vi "08-QNET_MECHKIT_Magnetic_Field.vi"() -> ()   [LabVIEW 2012]
doc: "This VI is to be used with the NI-ELVIS and the QNET-Mechatronic Sensors I module. The objective is to calibrate the magnetic field sensor."
uses:
  <vilib>/Simulation/Scripting/Companion Diagram/SimConfigNode/SimParams.ctl
  <vilib>/Simulation/Scripting/Companion Diagram/SimConfigNode/_simSolvers.ctl
  <vilib>/Simulation/Implementation/Shared/SIMSCR Execution Mode.ctl
  <vilib>/Simulation/Param Hierarchy/Typedefs/SIMPH Param Control Actions.ctl
  <vilib>/Simulation/Implementation/Shared/NILVSim_ParamChanged.vi
  <vilib>/Simulation/SignalDisplay/Implementation/NILVSim Time Waveform.llb/SIM Time Waveform (scalar).vi
  <vilib>/Simulation/Utility/Implementation/SIM Halt.vi
  <vilib>/Simulation/Implementation/Shared/NILVSim_Manager.vi
  <vilib>/Simulation/Implementation/Shared/NILVSim_FinalizeModel.vi
  <vilib>/Simulation/Implementation/Shared/SIM Unbundle Sim Info.vi
  <vilib>/Utility/error.llb/Clear Errors.vi
  <vilib>/Simulation/Implementation/Shared/NILVSim_GetModelError.vi
  <vilib>/Simulation/Implementation/Shared/SIM Bundle Sim Info.vi
  <vilib>/Simulation/Implementation/Shared/SIMSH Read Queue.vi
  <vilib>/Simulation/Implementation/Shared/NILVSim_Initialize.vi
  <vilib>/Analysis/6fits.llb/Unconstrained Exponential Fit.vi
  <vilib>/DAQmx/read.llb/DAQmx Read.vi
  <vilib>/DAQmx/read.llb/DAQmx Read (Analog DBL 1Chan 1Samp).vi
  <vilib>/Simulation/Utility/Implementation/NILVSim Get Time and IsAcceptedStep.vi
  <vilib>/Simulation/Scripting/Companion Diagram/SimConfigNode/SimDog.xnode
  <vilib>/Simulation/Implementation/XNodeFramework/SimXNode/SimX.xnode
  <vilib>/Analysis/NI_AALPro.lvlib
  <vilib>/Simulation/Implementation/Shared/NI_SIM_Implementation.lvlib
panel:
  in  "Sampling Rate (Hz)":dbl=100.0 min=0.0 max=1000.0 step=25.0 format="%.1f"
  in  "Device":tag="Dev1"
  in  "Tab Control":enum32{"Collect Data", "Calibrate Sensor"}(tab)
  out "Magnetic Field Sensor (V)":waveform(dbl)(graph)
  in  "Target Range (inch)":dbl[](array[numeric])
  in  "Sensor Measurement (V)":dbl[](array[numeric])
  out "Sensor Readings":T1(graph)
  out "a":dbl format="%#_3g"
  out "b":dbl format="%#_3g"
  out "Display: Magnetic Field (in)":dbl(slide) scale=0.0..0.5
  out "Magnetic Field (inch)":waveform(dbl)(graph)
  in  "Amplitude":dbl
  in  "Damping":dbl
  in  "stop":bool
  # "QNET-MECHKIT Magnetic Field"
  # "NOTE: Place J8 jumper on \"Magnetic Field\" setting."
  # "1) Rotate knob to change the target distance.\n2) Enter distance between opto sensor and target in \"Target Position (in)\" array.\n3) Enter measured sensor values in \"Sensor Measurement (V)\" array."
  # "Exponential curve fitting results:"
  # "y = a*exp(b*x)"
  # "Enter exponential parameters to measure correct target distance \n(e.g. display below should read 0.25 inches when the target is 0.25 inches from the reference point)."
  # "y = a*exp(b*x)\nwhere\na is the amplitude\nb is the damping\nx is the sensor voltage \ny is the output in inches."
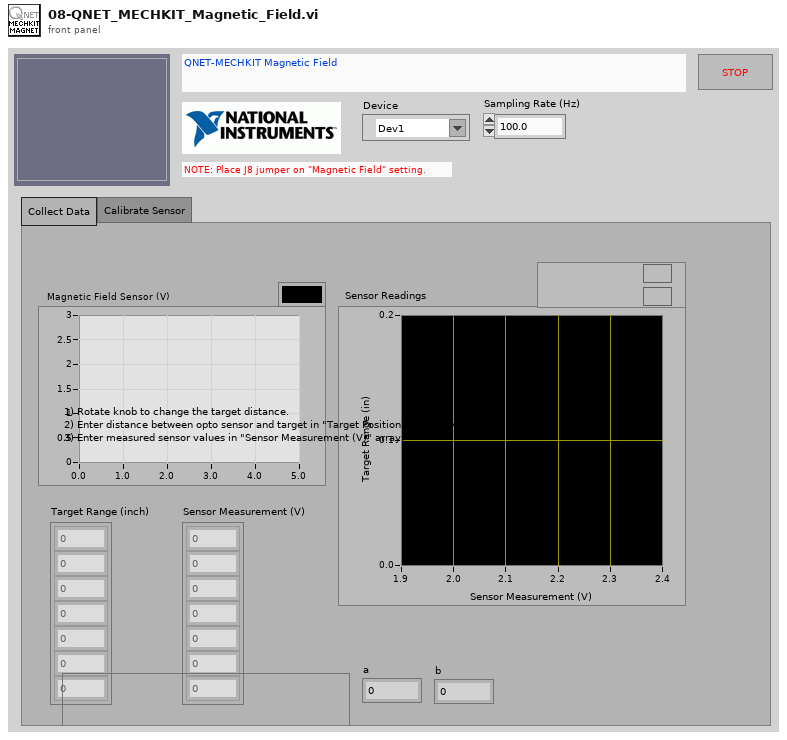
[diagram p1: front panel]
types:
  T1 = cluster{"Sensor Measurement (V)":dbl[], "Best Linear Fit":dbl[]}[]
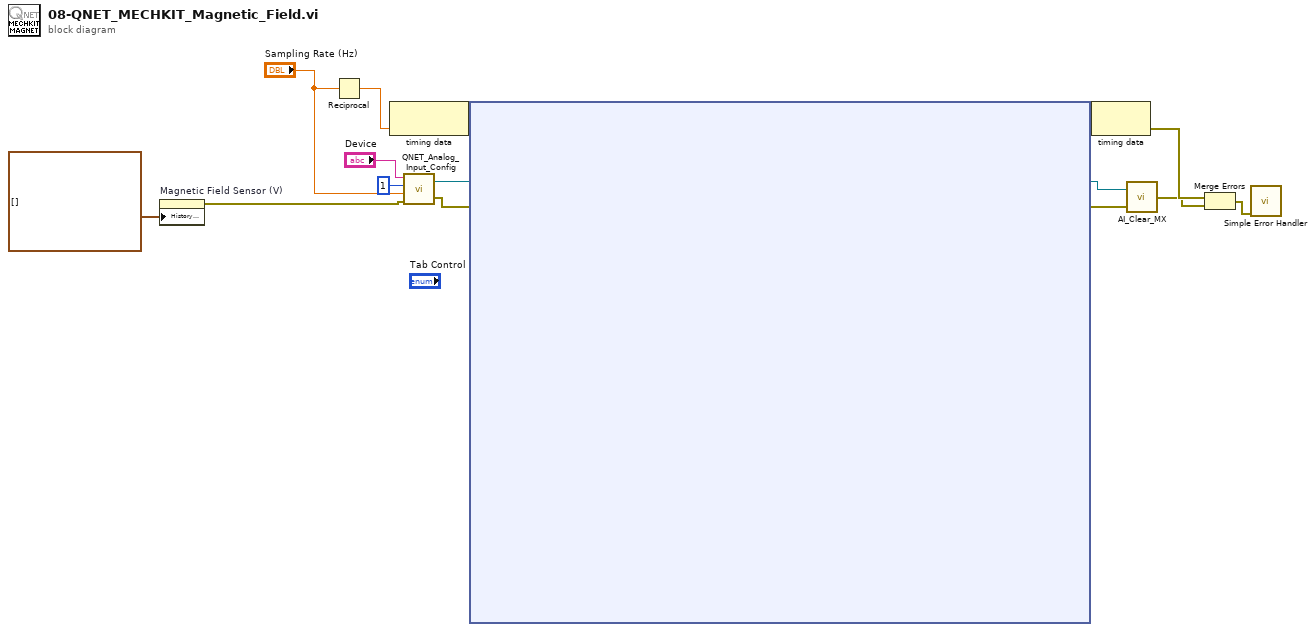
[diagram p0: block diagram]
diagram:
  n1 = property on="Magnetic Field Sensor (V)" class="WFChart (strict)"("History Data"=waveform(dbl)[] []) -> (error out=w2:errorcluster)  [unwired: 2 in, 1 out]
  n2 = Reciprocal(x="Sampling Rate (Hz)") -> (1/x=w6:dbl)
  n3 = node-c288(w6) -> (w14:variant)
  n4 = call "QNET_Analog_Input_Config.vi"("error in"=w2, "sampling rate (Hz)"="Sampling Rate (Hz)", "analog input channel"=u32 1, "dev"="Device") -> ("error out"=w11:errorcluster, "task out"=w10:refnum<k21>)
  n5 = node-c254 ("Simulation Loop")(w14, w11, w10) -> (w13:variant, w9:refnum<k21>, w8:errorcluster)
  n6 = node-c288(w13) -> (w5:errorcluster)
  n7 = call "AI_Clear_MX.vi"("Error in"=w8, "Task in"=w9) -> ("Error out"=w4:errorcluster)
  n8 = Merge Errors(w5, w4) -> (w3:errorcluster)
  n9 = call <vilib>:"Simple Error Handler.vi"("error in (no error)"=w3) -> ()  [unwired: 1 in, 8 out]
